vi "gfitsio-write-column-i32-1d.vi"(4 "units":string, 6 "row":i32, 7 "column":string, 8 "error in (no error)":errorcluster, 9 "data":i32[](array[numeric]), 10 "variable length? (T:yes)":bool=TRUE, 11 "gfits refnum":T1) -> (0 "error out":errorcluster, 3 "dup gfits refnum":T1)   [LabVIEW 2011, in "gfitsio.lvlib"]
doc: "Write data to the table column (doing data type conversion if necessary). This VI is not compatible with ASCII tables since ASCII tables can only contain scalar values columns."
uses:
  gfitsio.lvlib
  gfitsio-refnum.ctl
  cfitsio-hdutypes.ctl
  gfitsio.dll
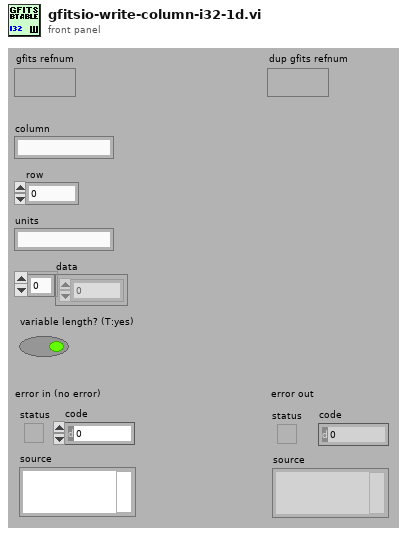
[diagram p1: front panel]
types:
  T1 = typedef "gfitsio.lvlib/gfitsio-refnum.ctl" = refnum<k1>
  T2 = typedef "gfitsio.lvlib/cfitsio-hdutypes.ctl" = i32
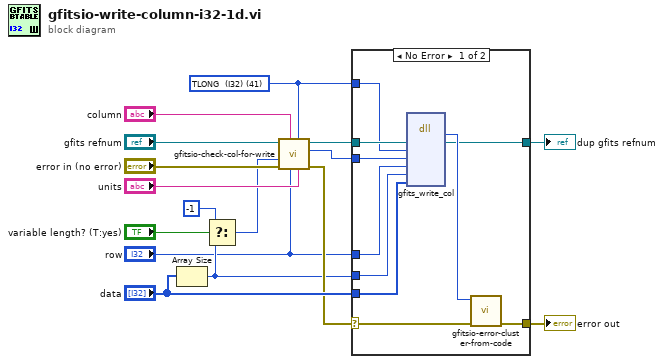
[diagram p0: block diagram]
diagram:
  w1 = T2 41 items=["TBIT"=1, "TBYTE  (U8)"=11, "TSBYTE  (I8)"=12, "TLOGICAL"=14, "TSTRING"=16, "TUSHORT  (U16)"=20, "TSHORT  (I16)"=21, "TUINT"=31, "TULONG  (U32)"=40, "TLONG  (I32)"=41, "TFLOAT  (SGL)"=42, "TLONGLONG  (I64)"=81, "TDOUBLE"=82, "TCOMPLEX  (CSG)"=83, "TDOUBLECOMPLEX  (CDB)"=163] ("cfitsio datatype")
  n1 = Array Size(array="data") -> (size(s)=w5:i32)
  n2 = Select(t=-1, s="variable length? (T:yes)", f=w5) -> (s? t:f=w4:i32)
  n3 = call "gfitsio-check-col-for-write.vi"("units"="units", "cfitsio datatype"=w1, "row"="row", "column"="column", "error in (no error)"="error in (no error)", "size (-1:variable)"=w4, "gfits refnum"="gfits refnum") -> ("error out"=w10:errorcluster, "colnum"=w7:i32, "dup gfits refnum"=w12:T1)  [unwired: 2 in]
  n4 = case shown="No Error" w10 {
    selector: w10 -> [w26 w28]
    tunnel: [w25 w28] -> w15
    tunnel: w12 -> [w19 w27]
    tunnel: [w23 w27] -> w16
    tunnel: "row" -> [w22 _]
    tunnel: "data" -> [w21 _]
    tunnel: w7 -> [w20 _]
    tunnel: w5 -> [w18 _]
    tunnel: w1 -> [w17 _]
    frame No Error {
      n5 = dll-call lib="C:/BonOMM/BonOMM-SAOMM/SubVIs/gfitsio/gfitsio.dll" fn="gfits_write_col"("dup gfits refnum"=w19, "datatype"=w17, "column"=w20, "row"=w22, "nelements"=w18, "data"=w21) -> (w24:i32, "dup gfits refnum"=w23:T1)  [unwired: 8 in, 2 out]
      n6 = call "gfitsio-error-cluster-from-code.vi"("error in (no error)"=w26, "error code"=w24) -> ("error out"=w25:errorcluster)  [unwired: 9 in]
    }
    frame Error {
    }
  }
  "error out" <- w15
  "dup gfits refnum" <- w16
